vi "Recall Bar Sample Resistivity Currents.vi"() -> (2 "Bar Sample Resistivity Currents":dbl[](array[numeric]))   [LabVIEW 2016, in "Hall Effect Library.lvlib"]
uses:
  Hall Effect Library.lvlib
  Private/Global Variables/Hall Effect Data.vi
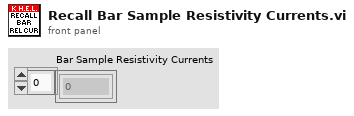
[diagram p1: front panel]
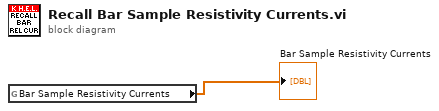
[diagram p0: block diagram]
diagram:
  n1 = global read "Hall Effect Data.vi" "Bar Sample Resistivity Currents"() -> (→"Bar Sample Resistivity Currents":dbl[])
